vi "Parse Push Refspecs.vi"(7 "All":bool, 8 "error in (no error)":errorcluster, 9 "Refspecs":string[](array[string]), 10 "Repository":string) -> (0 "error out":errorcluster, 3 "Final Argument String":string)   [LabVIEW 2017, in "Git-LabVIEW.lvlib" / "Git Implementation.lvclass"]
uses:
  Git Implementation.lvclass
  <vilib>/Utility/error.llb/whitespace.ctl
  <vilib>/Utility/error.llb/Error Cluster From Error Code.vi
  <vilib>/ErrorRing/Error Ring.xnode
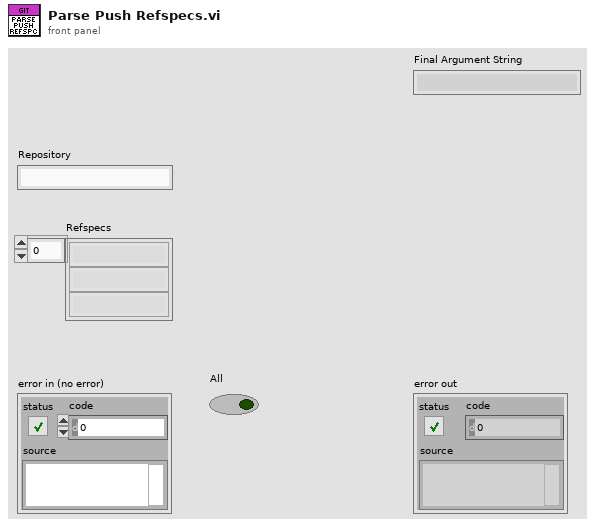
[diagram p1: front panel]
types:
  T1 = typedef "whitespace.ctl" = u16
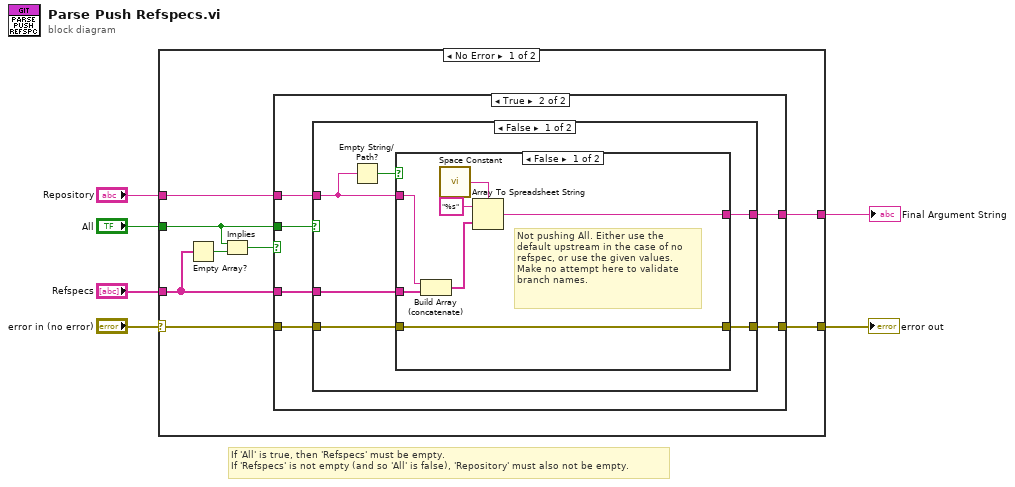
[diagram p0: block diagram]
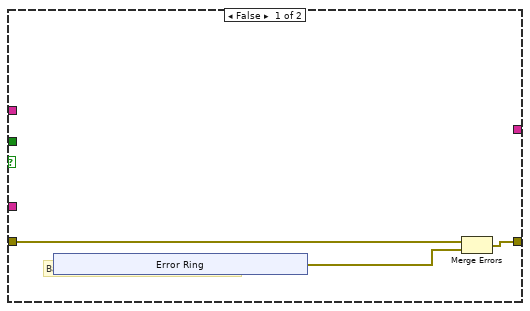
[diagram p2: hidden frame]
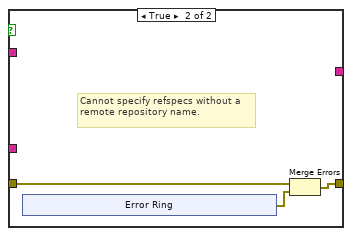
[diagram p3: hidden frame]
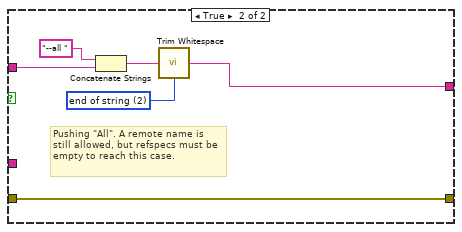
[diagram p4: hidden frame]
diagram:
  # "If 'All' is true, then 'Refspecs' must be empty.\nIf 'Refspecs' is not empty (and so 'All' is false), 'Repository' must also not be empty."
  n1 = case shown="No Error" "error in (no error)" {
    selector: "error in (no error)" -> [w12 w54]
    tunnel: [w11 w54] -> w5
    tunnel: "All" -> [w8 _]
    tunnel: "Repository" -> [w10 _]
    tunnel: "Refspecs" -> [w9 _]
    tunnel: [w7 _] -> w1
    frame No Error {
      n2 = Empty Array?(array=w9) -> (empty?=w14:bool)
      n3 = Implies(1:w14, 2:w8) -> (0:w13:bool)
      n4 = case shown="True" w13 {
        tunnel: w12 -> [w17 w23]
        tunnel: [w16 w24] -> w11
        tunnel: w10 -> [_ w26]
        tunnel: w9 -> [_ w22]
        tunnel: w8 -> [_ w27]
        tunnel: [_ w25] -> w7
        frame False {
          # "Bad combination of All and Refspecs"
          n5 = xnode "Error Ring"() -> ("error out"=w15:errorcluster)
          n6 = Merge Errors(w17, w15) -> (w16:errorcluster)
        }
        frame True {
          n7 = case shown="False" w27 {
            tunnel: w26 -> [w30 w52]
            tunnel: [w29 w49] -> w25
            tunnel: [w33 w50] -> w24
            tunnel: w23 -> [w32 w50]
            tunnel: w22 -> [w28 _]
            frame False {
              n8 = Empty String/Path?(string/path=w30) -> (empty?=w31:bool)
              n9 = case shown="False" w31 {
                tunnel: [w40 w41] -> w33
                tunnel: w32 -> [w40 w42]
                tunnel: w30 -> [w38 _]
                tunnel: [w34 _] -> w29
                tunnel: w28 -> [w39 _]
                frame False {
                  # "Not pushing All. Either use the default upstream in the case of no refspec, or use the given values.\nMake no attempt here to validate branch names."
                  n10 = Build Array (concatenate)(w38, w39) -> (w37:string[])
                  n11 = call <vilib>:"Space Constant.vi"() -> ("String"=w35:string)
                  n12 = Array To Spreadsheet String(delimiter (Tab)=w35, array=w37, 3:"%s" ("format string")) -> (spreadsheet string=w34:string)
                }
                frame True {
                  # "Cannot specify refspecs without a remote repository name."
                  n13 = xnode "Error Ring"() -> ("error out"=w43:errorcluster)
                  n14 = Merge Errors(w42, w43) -> (w41:errorcluster)
                }
              }
            }
            frame True {
              w48 = T1 2 items=["both", "start of string", "end of string"] ("location (both)")
              # "Pushing \"All\". A remote name is still allowed, but refspecs must be empty to reach this case."
              n15 = Concatenate Strings("--all ", w52) -> (w51:string)
              n16 = call <vilib>:"Trim Whitespace.vi"("string"=w51, "location (both)"=w48) -> ("trimmed string"=w49:string)
            }
          }
        }
      }
    }
    frame Error {
    }
  }
  "error out" <- w5
  "Final Argument String" <- w1
